vi "FRCts20_WebMethods_Documentation.vi"() -> ()   [LabVIEW 2014]
doc: "Generates documentation for all web methods."
uses:
  <vilib>/Utility/NIReport.llb/NI_ReportGenerationCore.lvlib
  <vilib>/Utility/NIReport.llb/NI_report.lvclass
  <vilib>/regexp/Match Regular Expression.xnode
  <vilib>/Utility/NIReport.llb/Append Report Text (str wrap).vi
  <vilib>/printing/ReportDocExtensions.llb/Append VI Icon to Report (path).vi
  <vilib>/printing/OpenHTMLReport.llb/Open HTML Report in Browser (Refnum).vi
  <vilib>/printing/ReportDocExtensions.llb/Append VI Description to Report (path).vi
panel:
  out "Slide":u8(slide) caption="Report Saved!" scale=0.0..100.0
  # "Note: Before running this VI make sure that you have read Append VI Description to Report (refnum).txt in the Utilities library and followed those instructions."
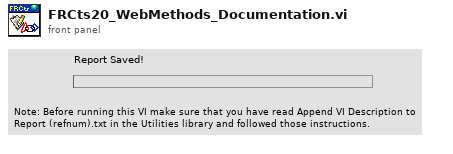
[diagram p1: front panel]
types:
  T1 = enum16{"Standard Report", "HTML", "Word", "Excel"}
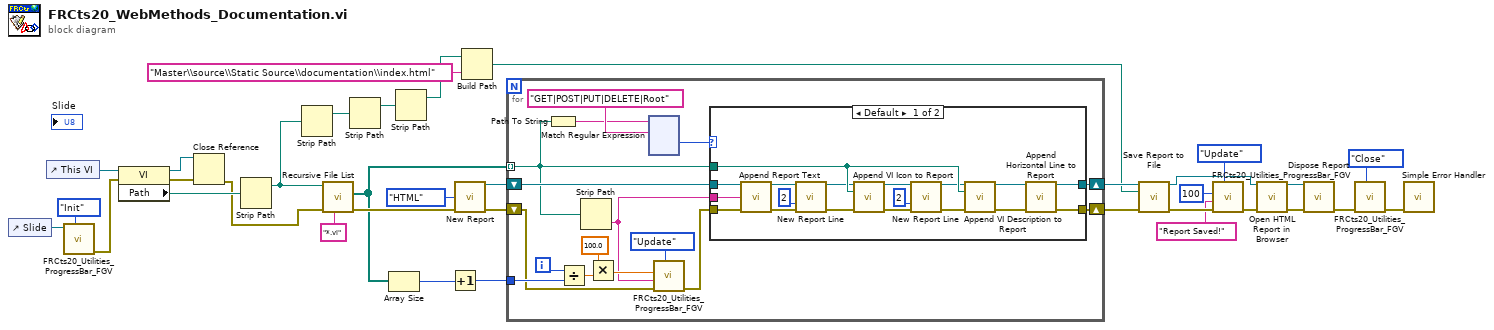
[diagram p0: block diagram]
diagram:
  n1 = control-ref of="Slide"() -> (w22:refnum<vi>)
  n2 = control-ref of="This VI"() -> (w35:refnum<vi>)
  n3 = call "FRCts20_Utilities_ProgressBar_FGV.vi"("Command"=enum16{"Close", "Update", "Init"}."Init", "Slide Reference"=w22) -> ("error out"=w21:errorcluster)  [unwired: 9 in]
  n4 = property class="VI"(reference=w35, error in=w21) -> (reference out=w31:refnum<vi>, error out=w32:errorcluster, "Path"=w34:path)
  n5 = Close Reference(reference=w31, error in (no error)=w32) -> (error out=w30:errorcluster)
  n6 = Strip Path(path=w34) -> (stripped path=w14:path)  [unwired: 1 out]
  n7 = Strip Path(path=w14) -> (stripped path=w13:path)  [unwired: 1 out]
  n8 = call <vilib>:"Recursive File List.vi"("pattern"="*.vi", "error in (no error)"=w30, "Folder Path"=w14) -> ("error out"=w28:errorcluster, "All Files in Dir"=w20:path[])  [unwired: 4 in, 3 out]
  n9 = Strip Path(path=w13) -> (stripped path=w12:path)  [unwired: 1 out]
  n10 = Array Size(array=w20) -> (size(s)=w8:i32)
  n11 = Strip Path(path=w12) -> (stripped path=w11:path)  [unwired: 1 out]
  n12 = Increment(x=w8) -> (x+1=w7:i32)
  n13 = call <vilib>:"New Report.vi"("report type"=T1."HTML", "error in (no error)"=w28) -> ("report out"=w26:refnum<class "NI_report.lvclass">, "error out"=w27:errorcluster)  [unwired: 12 in]
  n14 = Build Path(base path=w11, name or relative path="Master\\source\\Static Source\\documentation\\index.html") -> (appended path=w9:path)
  n15 = for {
    shift-right: [w51] -> w16
    shift-left: w27 -> [w42]
    tunnel: w20 -> [w37] mode=indexing
    shift-right: [w49] -> w15
    shift-left: w26 -> [w50]
    tunnel: w7 -> [w43]
    i -> [w44]
    n16 = Path To String(path=w37) -> (string=w41:string)
    n17 = Divide(x=w44, y=w43) -> (x/y=w39:dbl)
    n18 = Strip Path(path=w37) -> (name=w36:string)  [unwired: 1 out]
    n19 = Multiply(x=100.0 ("y"), y=w39) -> (x*y=w40:dbl)
    n20 = xnode "Match Regular Expression"("input string"=w41, "regular expression"="GET|POST|PUT|DELETE|Root") -> ("offset past match"=w48:i32)  [unwired: 4 in, 4 out]
    n21 = call "FRCts20_Utilities_ProgressBar_FGV.vi"("Command"=enum16{"Close", "Update", "Init"}."Update", "error in (no error)"=w42, "Text"=w36, "Percent"=w40) -> ("error out"=w46:errorcluster)  [unwired: 7 in]
    n22 = case shown="Default" w48 {
      tunnel: w37 -> [w180 _]
      tunnel: [w177 w181] -> w51
      tunnel: w46 -> [w171 w181]
      tunnel: w50 -> [w169 w182]
      tunnel: [w176 w182] -> w49
      tunnel: w36 -> [w170 _]
      frame Default {
        n23 = call-poly <vilib>:"Append Report Text.vi"("report in"=w169, "text"=w170, "error in (no error)"=w171) -> ("report out"=w168:refnum<class "NI_report.lvclass">, "error out"=w167:errorcluster)  [unwired: 9 in, 2 out]
        n24 = call-dynamic "New Report Line.vi"("report in"=w168, "number of lines (1)"=2, "error in (no error)"=w167) -> ("report out"=w165:refnum<class "NI_report.lvclass">, "error out"=w166:errorcluster)  [unwired: 11 in]
        n25 = call-poly <vilib>:"Append VI Icon to Report.vi"("report in"=w165, "VI"=w180, "error in (no error)"=w166) -> ("report out"=w175:refnum<class "NI_report.lvclass">, "error out"=w174:errorcluster)  [unwired: 8 in, 3 out]
        n26 = call-dynamic "New Report Line.vi"("report in"=w175, "number of lines (1)"=2, "error in (no error)"=w174) -> ("report out"=w172:refnum<class "NI_report.lvclass">, "error out"=w173:errorcluster)  [unwired: 11 in]
        n27 = call-poly <vilib>:"Append VI Description to Report.vi"("report in"=w172, "VI"=w180, "error in (no error)"=w173) -> ("report out"=w178:refnum<class "NI_report.lvclass">, "error out"=w179:errorcluster)  [unwired: 8 in, 3 out]
        n28 = call-dynamic "Append Horizontal Line to Report.vi"("report in"=w178, "error in (no error)"=w179) -> ("report out"=w176:refnum<class "NI_report.lvclass">, "error out"=w177:errorcluster)  [unwired: 12 in]
      }
      frame -1 {
        # "Not a web method"
      }
    }
  }
  n29 = call-dynamic "Save Report to File.vi"("report in"=w15, "report file path"=w9, "error in (no error)"=w16) -> ("report out"=w4:refnum<class "NI_report.lvclass">, "error out"=w2:errorcluster)  [unwired: 11 in]
  n30 = call "FRCts20_Utilities_ProgressBar_FGV.vi"("Command"=enum16{"Close", "Update", "Init"}."Update", "error in (no error)"=w2, "Text"="Report Saved!", "Percent"=u8 100) -> ("error out"=w5:errorcluster)  [unwired: 7 in]
  n31 = call-poly <vilib>:"Open HTML Report in Browser.vi"("report in"=w4, "error in (no error)"=w5) -> ("report out"=w24:refnum<class "NI_report.lvclass">, "error out"=w25:errorcluster)  [unwired: 11 in, 1 out]
  n32 = call-dynamic "Dispose Report.vi"("report in"=w24, "error in (no error)"=w25) -> ("error out"=w19:errorcluster)  [unwired: 13 in]
  n33 = call "FRCts20_Utilities_ProgressBar_FGV.vi"("Command"=enum16{"Close", "Update", "Init"}."Close", "error in (no error)"=w19) -> ("error out"=w18:errorcluster)  [unwired: 9 in]
  n34 = call <vilib>:"Simple Error Handler.vi"("error in (no error)"=w18) -> ()  [unwired: 4 in, 5 out]
